vi "Main_Continuous.vi"() -> ()   [LabVIEW 2017]
doc: "This sample project is built upon the standard state machine template and shows how you could create an application that acquires, analyzes, and presents data. It includes functionality for presenting configuration dialogs, preserving settings between executions, loading and saving data, as well as exporting graph images and text files.\n\nIt is most appropriate for data that is acquired instantly as it does not allow for screen updates mid acquisition nor does it allow for continuous streaming to disk."
uses:
  controls/State.ctl
  controls/Data.ctl
  <vilib>/Utility/miscctls.llb/LVCursorListTypeDef.ctl
  <vilib>/Utility/miscctls.llb/LVAnnotationListTypeDef.ctl
  controls/UI References.ctl
  controls/HW Configuration.ctl
  controls/New Data Behavior.ctl
  controls/User Specified Data.ctl
  controls/Graph Data.ctl
  controls/Analysis Configuration.ctl
  subVIs/Settings Dialog.vi
  <extravilib>/ChannelInstances/Event Messenger-str.lvlib
  original/controls/Simulated Signal Type.ctl
  Program Files/National Instruments/LabVIEW 2017/examples/Data Communication/Protocols/TCP/TCP Multiple Connections/controls/TCP Multiple Connections State.ctl
  Program Files/National Instruments/LabVIEW 2017/examples/Data Communication/Protocols/TCP/TCP Multiple Connections/controls/TCP Multiple Connections Data.ctl
  <extravilib>/ChannelInstances/Event Messenger-c(a[.](str),t'Data.ctl').lvlib
  <extravilib>/ChannelInstances/Stream-t'Data.ctl'.lvlib
  controls/Signal Configuration.ctl
panel:
  out "# of Connections":i32
  in  "Settings":bool
  in  "Snapshot":bool
  in  "Analyze":bool
  in  "Clear":bool
  in  "Exit":bool
  in  "Acquire":bool
  in  "Export":bool
  in  "Save Data":bool
  in  "Load Data":bool
  out "Graph":waveform(dbl)[](graph)
  out "Status Bar":string
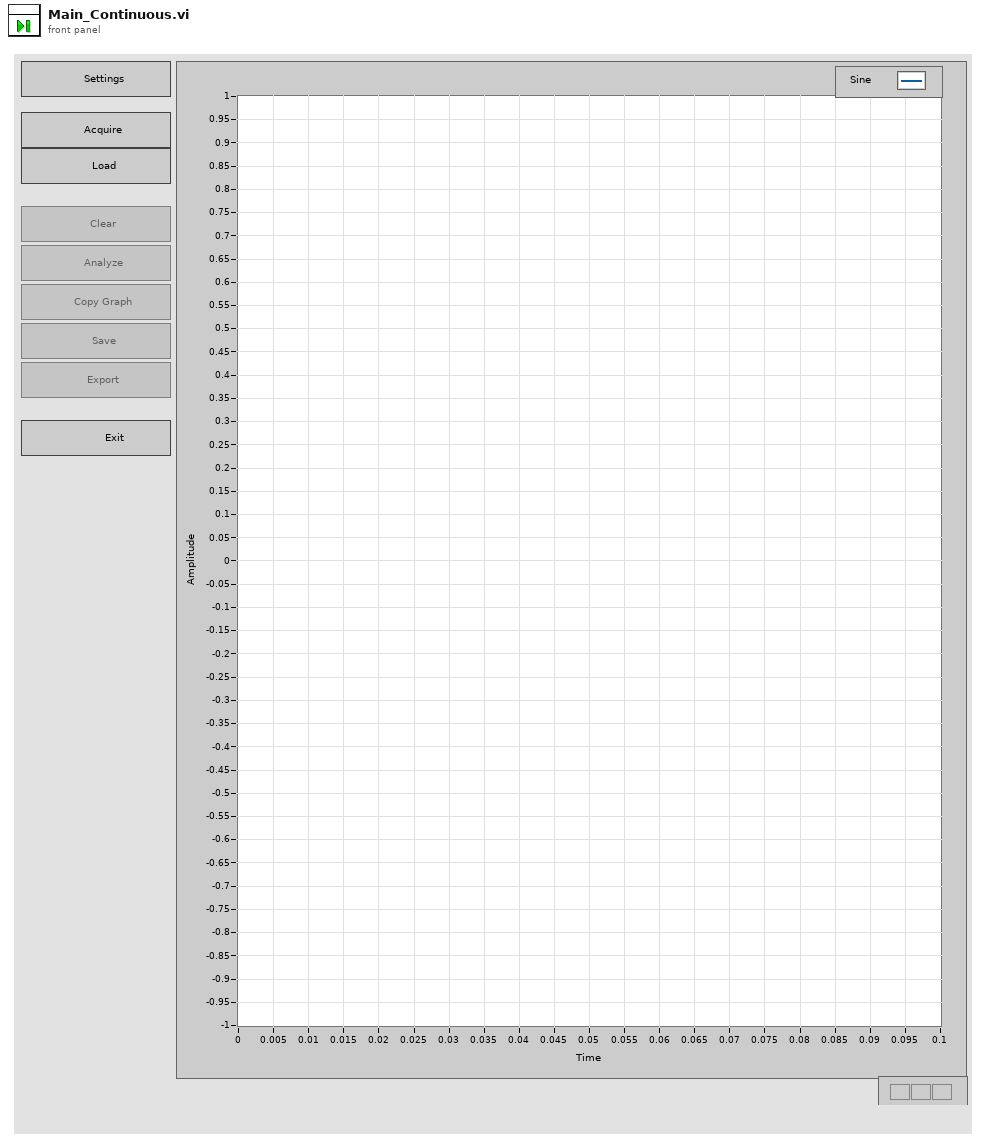
[diagram p1: front panel]
types:
  T1 = typedef "TCP Multiple Connections Data.ctl" = cluster{"Clients":refnum<k5>[], "Listener":refnum<k5>}
  T2 = typedef "TCP Multiple Connections State.ctl" = enum16{"Initialize", "Status Check", "Send Data", "Stop"}
  T3 = typedef "Data.ctl" = cluster{"UI References":T4, "Graph Data":T5, "User Specified":T8}
  T4 = typedef "UI References.ctl" = cluster{"Exit Ref":refnum<vi>, "Save Ref":refnum<vi>, "Open Ref":refnum<vi>, "Export Ref":refnum<vi>, "Acquire Ref":refnum<vi>, "Configure Ref":refnum<vi>, "Graph Ref":refnum<vi>, "Clear Ref":refnum<vi>, "Analyze Ref":refnum<vi>, "Status Ref":refnum<vi>, "Snapshot Ref":refnum<vi>}
  T5 = typedef "Graph Data.ctl" = cluster{"Data":waveform(dbl)[], "Annotation List":T6, "Cursor List":T7, "Analysis Data":waveform(dbl)[]}
  T6 = typedef "LVAnnotationListTypeDef.ctl" = cluster{"Name":string, "Color":u32, "Style":u8, "Point Style":u8, "Name Visible":bool, "Allow Drag":bool, "Annotation Mode":u32, "Plot":i32, "Index":i32, "Position":cluster{"X":dbl, "Y":dbl}, "X Scale":u32, "Y Scale":u32, "Show Arrow":bool, "Lock Name":bool, "Plot Area":i32, "Label Offset":cluster{"X":dbl, "Y":dbl}}[]
  T7 = typedef "LVCursorListTypeDef.ctl" = cluster{"Name":string, "Color":u32, "Style":u8, "Point Style":u8, "Name Visible":bool, "Allow Drag":bool, "Cursor Mode":u32, "Plot":i32, "Index":i32, "Position":cluster{"X":dbl, "Y":dbl}, "X Scale":u32, "Y Scale":u32, "Watch Plots":i32[], "Watch All Plots":bool, "Plot Area":i32, "Label Offset":cluster{"X":dbl, "Y":dbl}}[]
  T8 = typedef "User Specified Data.ctl" = cluster{"Hardware Configuration":T9, "Analysis Configuration":T11, "Signal Type":enum16{"Single Chirp", "From Excel"}, "New Data Behavior":T12, "Signal Configuration":T13}
  T9 = typedef "HW Configuration.ctl" = cluster{"Signal Channel":tag, "Response Channel":tag, "Trigger Channel":tag, "HW Refnum <Replace Me>":string, "Signal Type <Replace Me>":T10}
  T10 = typedef "Simulated Signal Type.ctl" = enum16{"Sine Wave", "Square Wave"}
  T11 = typedef "Analysis Configuration.ctl" = cluster{"Statistics":bool}
  T12 = typedef "New Data Behavior.ctl" = enum16{"Replace", "Overlay", "Append"}
  T13 = typedef "Signal Configuration.ctl" = cluster{"Chirp Amplitude":dbl, "I/O Limit":dbl, "Sample Rate":dbl, "Chirp Duration (s)":dbl, "Upper Frequency":dbl, "Lower Frequency":dbl, "Windowing":enum16{"None", "Exponential", "Flat top", "Hamming", "Hanning", "Kaiser-Bessel", "Rectangular"}}
  T14 = typedef "State.ctl" = enum16{"Initialize", "Wait for Event", "Update UI", "Configure", "Acquire", "Load Data", "Save Data", "Clear Data", "Export Data", "Analyze", "Copy Graph", "Exit"}
  T15 = enum16{"Standard", "Buffered", "CRLF", "Immediate"}
  T16 = typedef "Event Messenger-str.lvlib/))Channel.ctl" = refnum<queue>
  T17 = typedef "Event Messenger-c(a[.](str),t'Data.ctl').lvlib/))Channel.ctl" = refnum<queue>
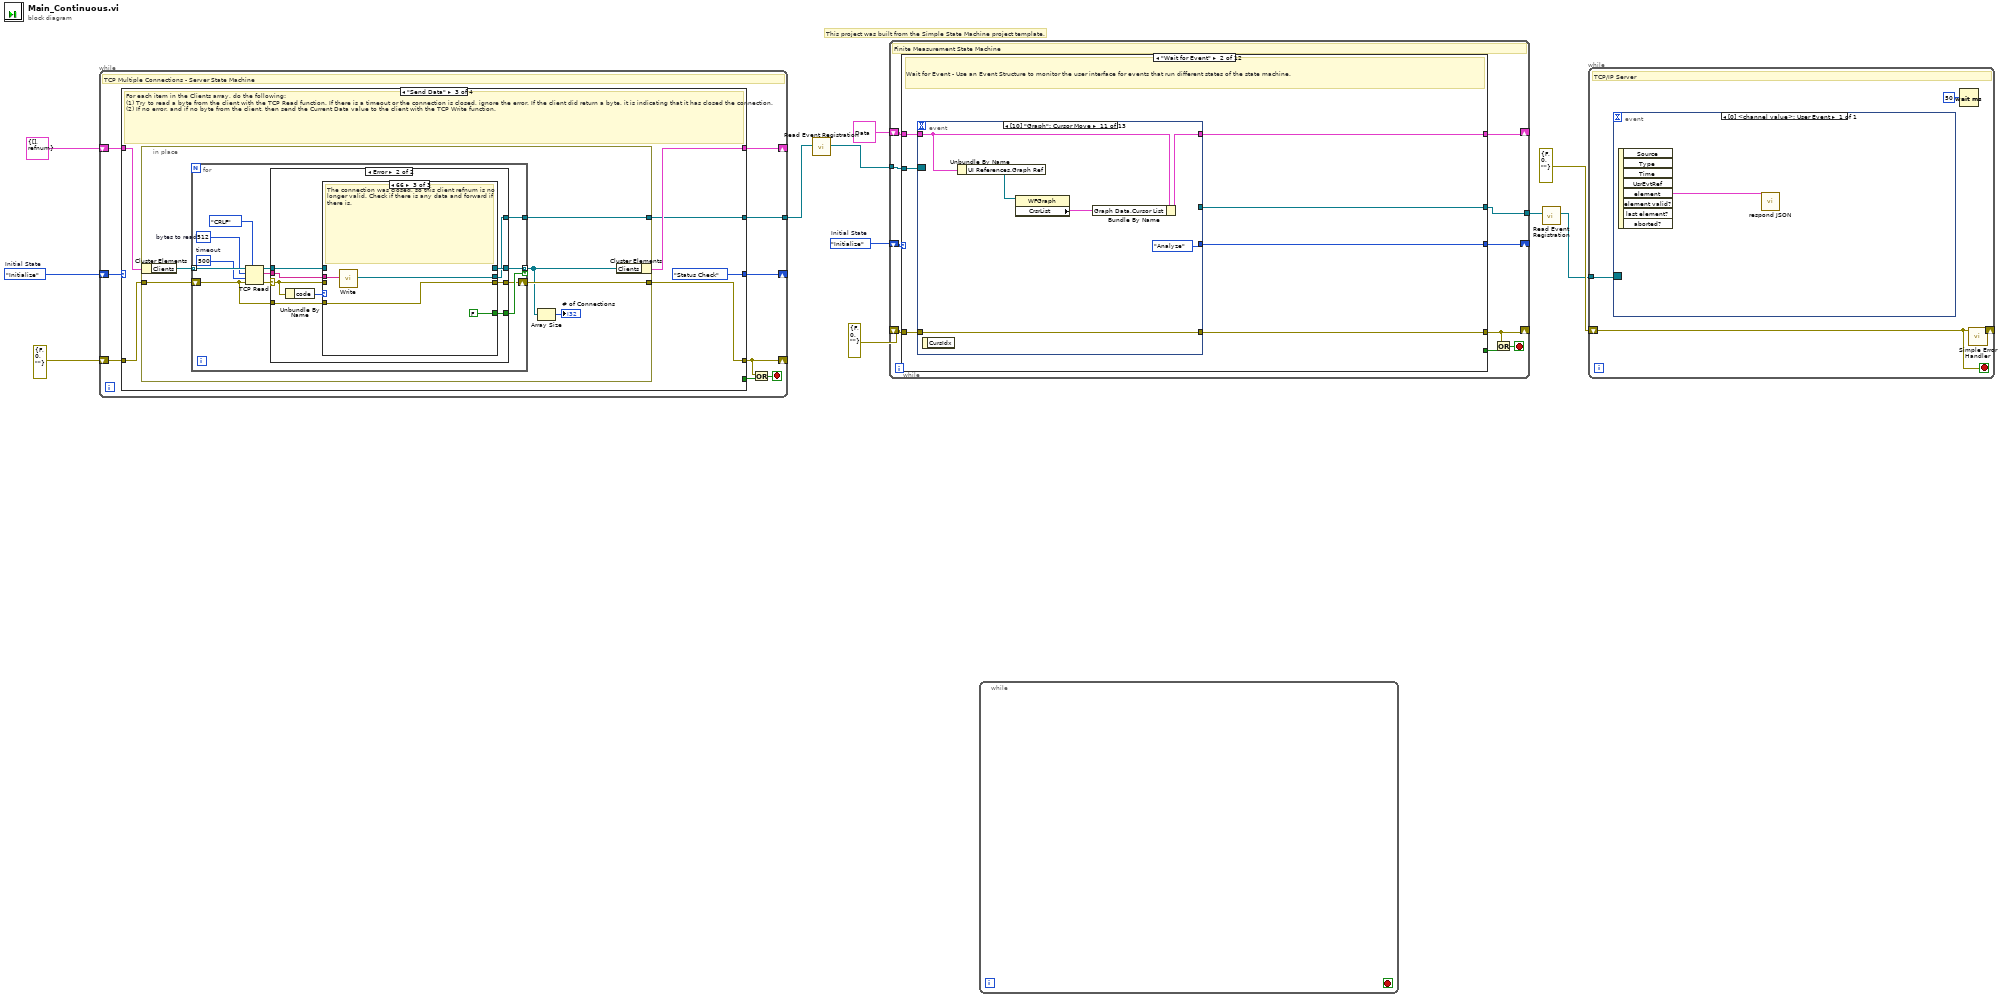
[diagram p0: block diagram]
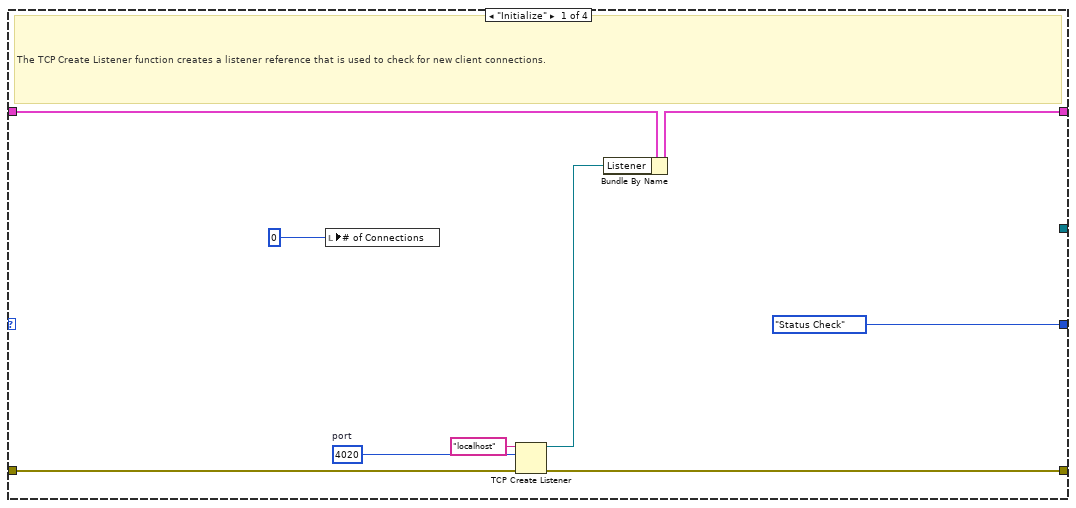
[diagram p2: hidden frame]
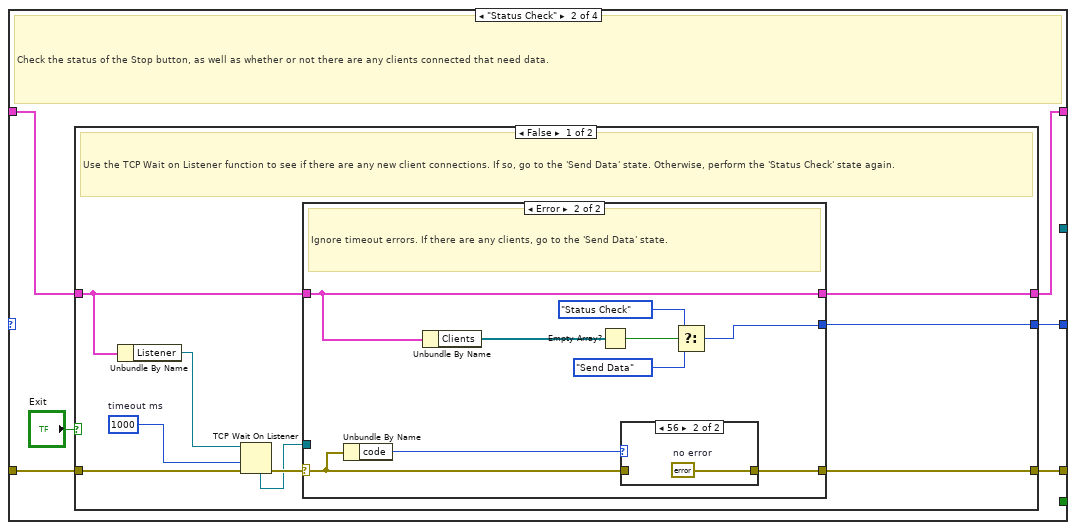
[diagram p3: hidden frame]
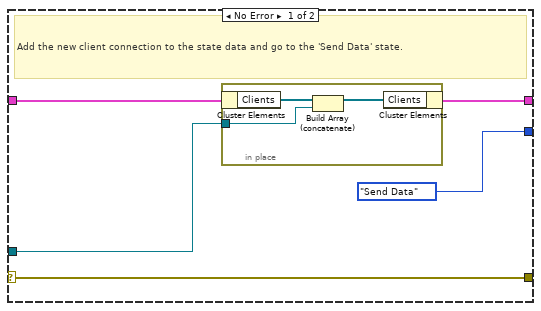
[diagram p4: hidden frame]
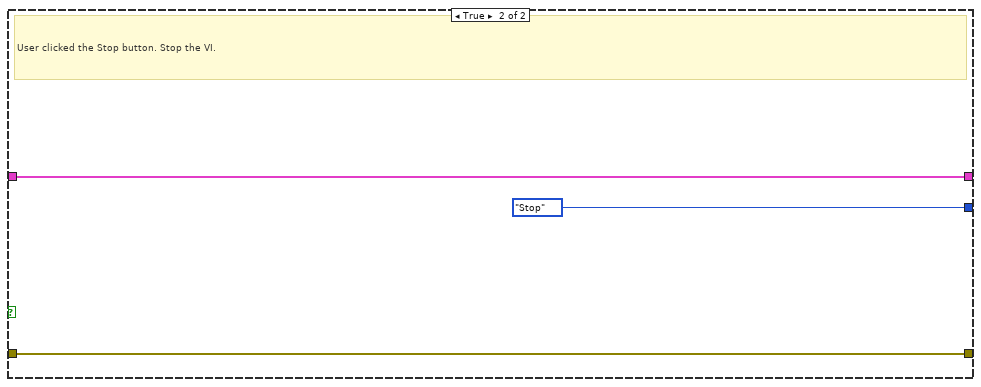
[diagram p6: hidden frame]
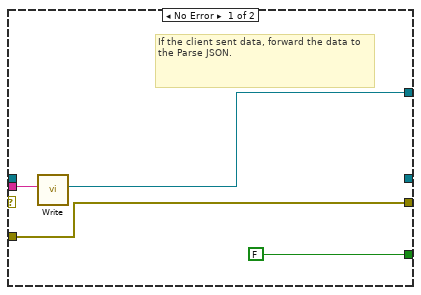
[diagram p7: hidden frame]
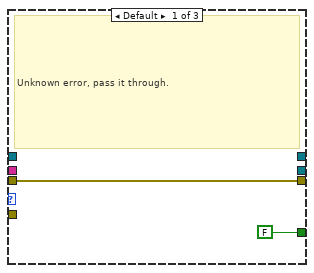
[diagram p8: hidden frame]
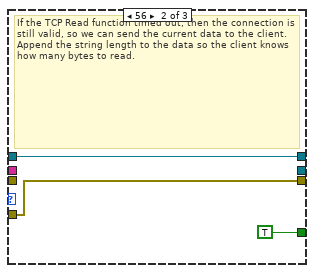
[diagram p9: hidden frame]
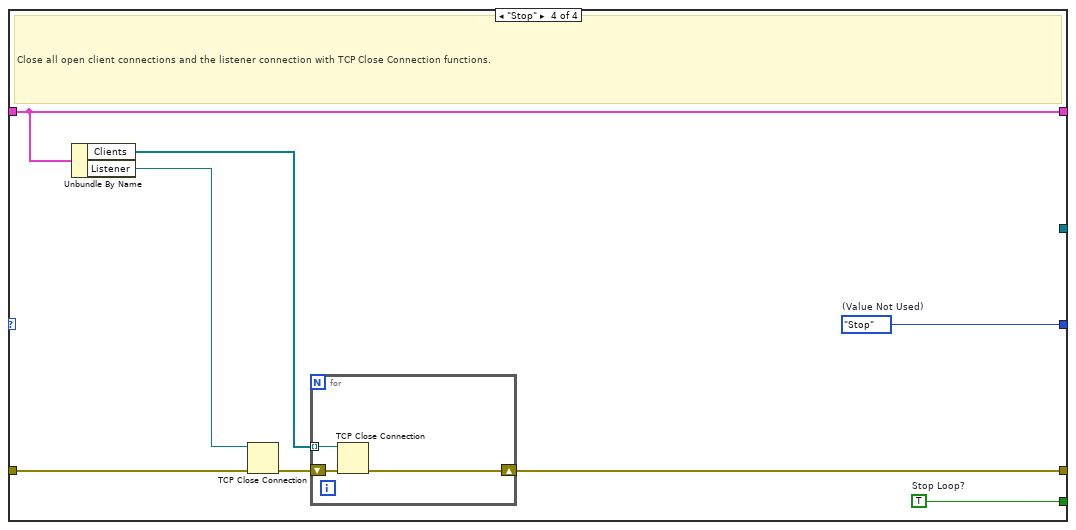
[diagram p10: hidden frame]
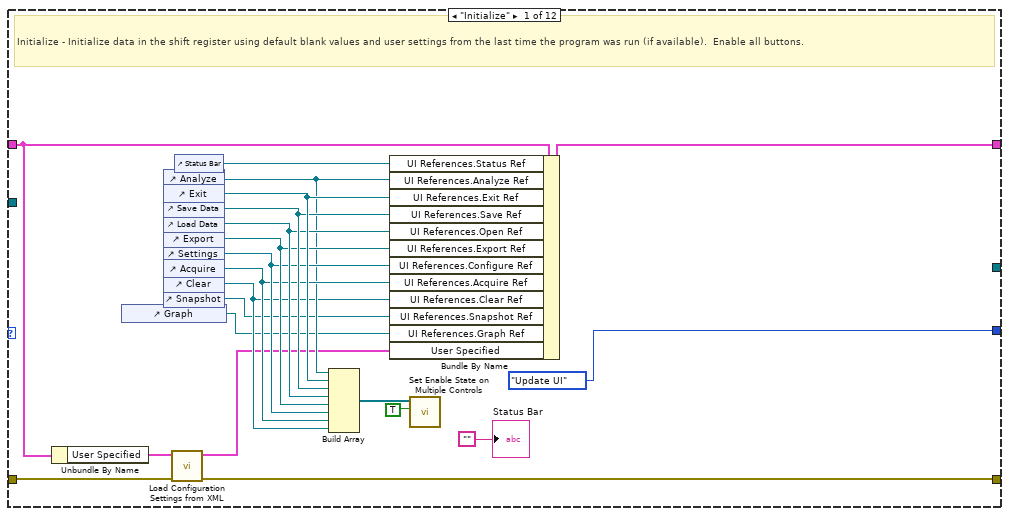
[diagram p11: hidden frame]
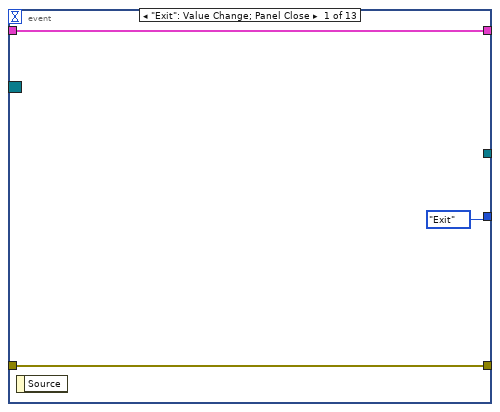
[diagram p12: hidden frame]
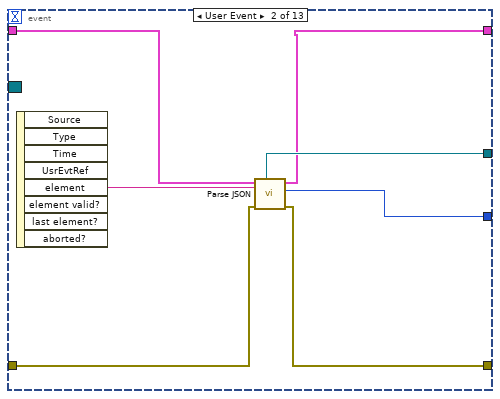
[diagram p13: hidden frame]
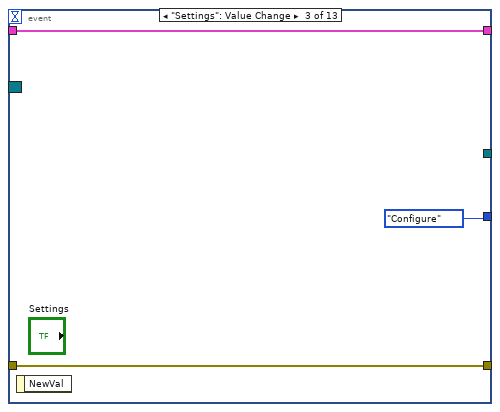
[diagram p14: hidden frame]
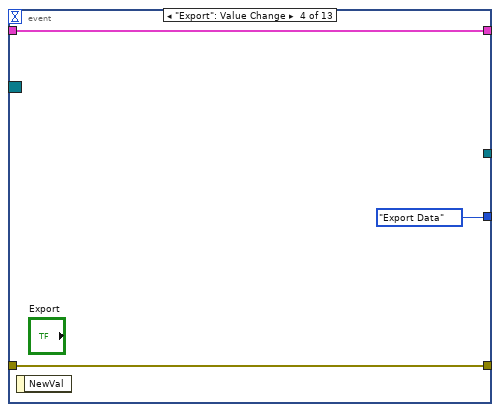
[diagram p15: hidden frame]
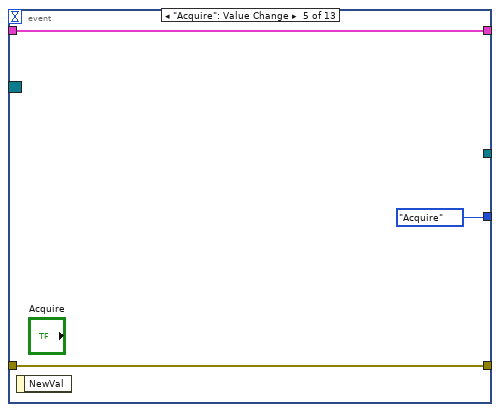
[diagram p16: hidden frame]
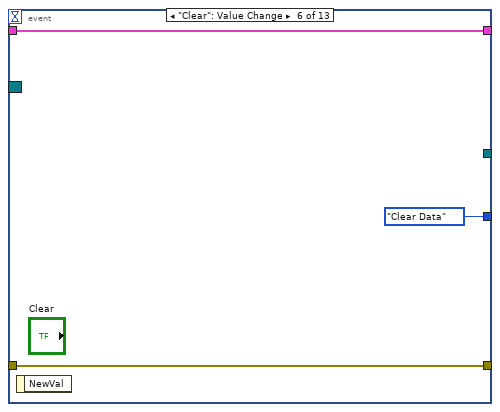
[diagram p17: hidden frame]
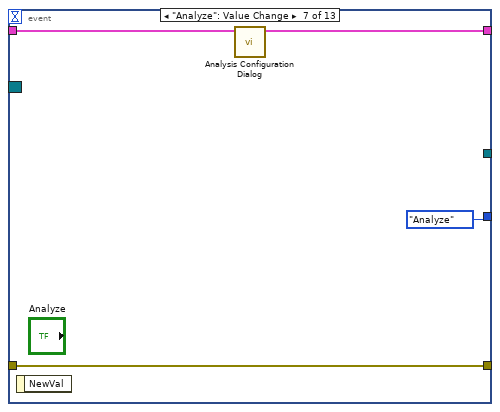
[diagram p18: hidden frame]
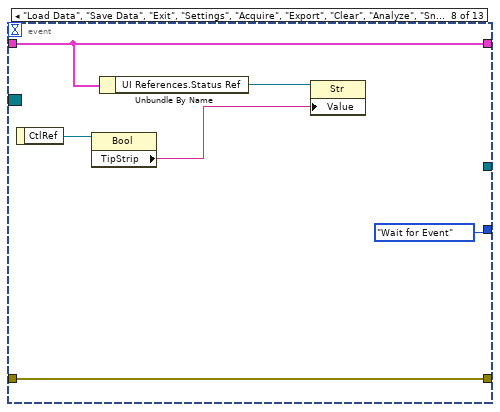
[diagram p19: hidden frame]
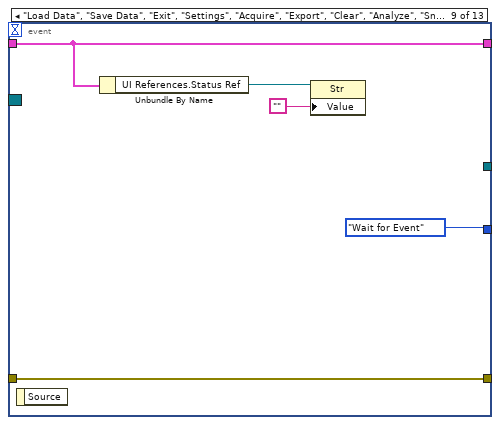
[diagram p20: hidden frame]
diagram:
  w4 = TCP_Multiple_Connections_State."Initialize"  # Initial State
  w11 = State."Initialize"  # Initial State
  # "This project was built from the Simple State Machine project template."
  n1 = while {
    shift-right: [w19] -> _
    shift-left: w4 -> [w20]
    shift-right: [w17] -> _
    shift-left: T1 {"Clients"=[], "Listener"=refnum} ("Data") -> [w18]
    shift-right: [w13] -> _
    shift-left: errorcluster {"status"=FALSE, "code"=0, "source"=""} ("error constant") -> [w16]
    tunnel: [w12] -> w1
    stop <- w14 stop-if-true
    # "TCP Multiple Connections - Server State Machine"
    n2 = case shown="\"Send Data\"" w20 {
      tunnel: [TCP_Multiple_Connections_State."Status Check" ("States") w35 TCP_Multiple_Connections_State."Status Check" ("States") w113] -> w19
      tunnel: [_ _ _ w120] -> w15
      tunnel: w18 -> [w27 w32 w70 w119]
      tunnel: [w26 w31 w69 w119] -> w17
      tunnel: w16 -> [w29 w34 w72 w118]
      tunnel: [w28 w33 w71 w116] -> w13
      tunnel: [_ _ w67 _] -> w12
      frame "Initialize" {
        w24 = u16 4020  # port
        # "The TCP Create Listener function creates a listener reference that is used to check for new client connections."
        n3 = local write "# of Connections"(0 ("Number of Client Connections")) -> ()
        n4 = TCP Create Listener(8:w29, 10:w24, 11:"localhost" ("service name")) -> (0:w28:errorcluster, 3:w25:refnum<k5>)  [unwired: 3 out]
        n5 = Bundle By Name(cluster=w27, "Listener"=w25) -> (w26:T1)
      }
      frame "Status Check" {
        # "Check the status of the Stop button, as well as whether or not there are any clients connected that need data."
        n6 = case shown="False" "Exit" {
          tunnel: [w44 TCP_Multiple_Connections_State."Stop" ("States")] -> w35
          tunnel: w34 -> [w43 w66]
          tunnel: [w36 w66] -> w33
          tunnel: w32 -> [w39 w65]
          tunnel: [w38 w65] -> w31
          frame False {
            w42 = 1000  # timeout ms
            # "Use the TCP Wait on Listener function to see if there are any new client connections. If so, go to the 'Send Data' state. Otherwise, perform the 'Status Check' state again."
            n7 = Unbundle By Name(w39) -> ("Listener"=w37:refnum<k5>)
            n8 = TCP Wait On Listener(8:w43, 9:w42, 11:w37) -> (0:w41:errorcluster, 4:w40:refnum<k5>)  [unwired: 4 out]
            n9 = case shown="Error" w41 {
              selector: w41 -> [w47 w61]
              tunnel: [TCP_Multiple_Connections_State."Send Data" ("States") w55] -> w44
              tunnel: w40 -> [w48 _]
              tunnel: w39 -> [w49 w58]
              tunnel: [w46 w58] -> w38
              tunnel: [w47 w59] -> w36
              frame No Error {
                # "Add the new client connection to the state data and go to the 'Send Data' state."
                n10 = in-place {
                  in-place-border: w48 -> [w50]
                  n11 = in-place-cluster #1(w49) -> ("Clients"=w52:refnum<k5>[])
                  n12 = Build Array (concatenate)(w52, w50) -> (w51:refnum<k5>[])
                  n13 = in-place-cluster #1("Clients"=w51) -> (w46:T1)
                }
              }
              frame Error {
                # "Ignore timeout errors. If there are any clients, go to the 'Send Data' state."
                n14 = Unbundle By Name(w61) -> ("code"=w60:i32)
                n15 = Unbundle By Name(w58) -> ("Clients"=w57:refnum<k5>[])
                n16 = Empty Array?(array=w57) -> (empty?=w56:bool)
                n17 = case shown="56" w60 {
                  tunnel: w61 -> [w62 _]
                  tunnel: [w62 w63] -> w59
                  frame Default {
                  }
                  frame 56 {
                    w63 = errorcluster {"status"=FALSE, "code"=0, "source"=""}  # no error
                  }
                }
                n18 = Select(t=TCP_Multiple_Connections_State."Status Check" ("States"), s=w56, f=TCP_Multiple_Connections_State."Send Data" ("States")) -> (s? t:f=w55:T2)
              }
            }
          }
          frame True {
            # "User clicked the Stop button. Stop the VI."
          }
        }
      }
      frame "Send Data" {
        # "For each item in the Clients array, do the following:\n(1) Try to read a byte from the client with the TCP Read function. If there is a timeout or the connection is closed, ignore the error. If the client did return a byte, it is indicating that it has closed the connection.\n(2) If no error, and if no byte from the client, then send the Current Data value to the client with the TCP Write function."
        n19 = in-place {
          in-place-border: w72 -> [w78]
          in-place-border: [w77] -> w71
          in-place-border: [w73] -> w67
          n20 = in-place-cluster #2(w70) -> ("Clients"=w75:refnum<k5>[])
          n21 = for {
            tunnel: w75 -> [w90] mode=indexing
            shift-right: [w82] -> w77
            shift-left: w78 -> [w81]
            tunnel: [w84] -> w74 mode=indexing if=w83
            tunnel: [w79] -> w73
            w87 = 500  # timeout
            w88 = 512  # bytes to read
            n22 = TCP Read(connection ID=w90, bytes to read=w88, error in (no error)=w81, 7:T15."CRLF" ("mode (standard)"), 9:w87) -> (connection ID out=w89:refnum<k5>, data out=w85:string, error out=w86:errorcluster)
            n23 = case shown="Error" w86 {
              selector: w86 -> [_ w102]
              tunnel: w89 -> [_ w99]
              tunnel: w85 -> [w93 w96]
              tunnel: [_ w97] -> w84
              tunnel: [FALSE w98] -> w83
              tunnel: [w91 w101] -> w82
              tunnel: w81 -> [w91 w100]
              tunnel: [w92 w95] -> w79
              frame No Error {
                # "If the client sent data, forward the data to the Parse JSON."
                # "If the client sent data, it is saying that the connection should be closed."
                n24 = call <extravilib>:"Write.vi"("element"=w93) -> ("channel"=w92:T16)  [unwired: 9 in, 1 out]
              }
              frame Error {
                # "Ignore connection closed and timeout errors"
                n25 = Unbundle By Name(w102) -> ("code"=w103:i32)
                n26 = case shown="66" w103 {
                  tunnel: w102 -> [w105 _ _]
                  tunnel: [w105 w106 w112] -> w101
                  tunnel: w100 -> [_ w106 w112]
                  tunnel: w99 -> [_ w108 _]
                  tunnel: [FALSE TRUE FALSE] -> w98
                  tunnel: [_ w108 _] -> w97
                  tunnel: w96 -> [_ _ w110]
                  tunnel: [_ _ w109] -> w95
                  frame Default {
                    # "Unknown error, pass it through."
                  }
                  frame 56 {
                    # "If the TCP Read function timed out, then the connection is still valid, so we can send the current data to the client. Append the string length to the data so the client knows how many bytes to read."
                  }
                  frame 66 {
                    # "The connection was closed, so this client refnum is no longer valid. Check if there is any data and forward if there is."
                    n27 = call <extravilib>:"Write.vi"("element"=w110) -> ("channel"=w109:T16)  [unwired: 9 in, 1 out]
                  }
                }
              }
            }
          }
          n28 = Array Size(array=w74) -> (size(s)=→"# of Connections":i32)
          n29 = in-place-cluster #2("Clients"=w74) -> (w69:T1)
        }
      }
      frame "Stop" {
        w113 = TCP_Multiple_Connections_State."Stop"  # (Value Not Used)
        w120 = TRUE  # Stop Loop?
        # "Close all open client connections and the listener connection with TCP Close Connection functions."
        n30 = Unbundle By Name(w119) -> ("Clients"=w117:refnum<k5>[], "Listener"=w114:refnum<k5>)
        n31 = TCP Close Connection(connection ID=w114, error in (no error)=w118) -> (error out=w115:errorcluster)  [unwired: 1 in, 1 out]
        n32 = for {
          shift-right: [w122] -> w116
          shift-left: w115 -> [w123]
          tunnel: w117 -> [w121] mode=indexing
          n33 = TCP Close Connection(connection ID=w121, error in (no error)=w123) -> (error out=w122:errorcluster)  [unwired: 1 in, 1 out]
        }
      }
    }
    n34 = Or(x=w13, y=w15) -> (x .or. y?=w14:bool)
  }
  n35 = call <extravilib>:"Read Event Registration.vi"("channel"=w1) -> ("event registration refnum"=w9:refnum<event-registration>)  [unwired: 10 in]
  n36 = while {
    shift-right: [w125] -> _
    shift-left: w11 -> [w133]
    shift-right: [w131] -> _
    shift-left: T3 {"UI References"={"Exit Ref"=refnum, "Save Ref"=refnum, "Open Ref"=refnum, "Export Ref"=refnum, "Acquire Ref"=refnum, "Configure Ref"=refnum, "Graph Ref"=refnum, "Clear Ref"=refnum, "Analyze Ref"=refnum, "Status Ref"=refnum, "Snapshot Ref"=refnum}, "Graph Data"={"Data"=[], "Annotation List"=[], "Cursor List"=[], "Analysis Data"=[]}, "User Specified"={"Hardware Configuration"={"Signal Channel"="", "Response Channel"="", "Trigger Channel"="", "HW Refnum <Replace Me>"="", "Signal Type <Replace Me>"=enum."Sine Wave"}, "Analysis Configuration"={"Statistics"=TRUE}, "Signal Type"=enum."Single Chirp", "New Data Behavior"=enum."Replace", "Signal Configuration"={"Chirp Amplitude"=0.1, "I/O Limit"=10.0, "Sample Rate"=1000000.0, "Chirp Duration (s)"=0.01, "Upper Frequency"=0.0, "Lower Frequency"=0.0, "Windowing"=enum."None"}}} ("Data") -> [w132]
    shift-right: [w128] -> _
    shift-left: errorcluster {"status"=FALSE, "code"=0, "source"=""} ("error constant") -> [w130]
    tunnel: w9 -> [w127]
    tunnel: [w126] -> w6
    stop <- w124 stop-if-true
    # "Finite Measurement State Machine"
    n37 = case shown="\"Wait for Event\"" w133 {
      tunnel: [_ w161 _ _ _ _ _ _ _ _ _ _] -> w126
      tunnel: [_ _ _ _ _ _ _ _ _ _ _ w321] -> w129
      tunnel: w132 -> [w146 w160 w229 w241 w242 w267 w281 w293 w304 w307 w313 w319]
      tunnel: [w154 w159 w229 w240 w249 w262 w281 w293 w303 w307 w313 w319] -> w131
      tunnel: w130 -> [w144 w158 w231 w239 w250 w266 w283 w296 w305 w308 w312 w316]
      tunnel: [w143 w157 w231 w238 w250 w265 w279 w290 w305 w308 w311 w315] -> w128
      tunnel: w127 -> [_ w156 _ _ _ _ _ _ _ _ _ _]
      tunnel: [State."Update UI" ("Next State") w155 State."Wait for Event" ("(Value Not Used)") w232 State."Update UI" ("Next State") State."Update UI" ("(Value Not Used)") State."Wait for Event" ("(Value Not Used)") State."Wait for Event" ("(Value Not Used)") State."Update UI" ("(Value Not Used)") State."Update UI" ("(Value Not Used)") State."Wait for Event" ("(Value Not Used)") w314] -> w125
      frame "Initialize" {
        # "Initialize - Initialize data in the shift register using default blank values and user settings from the last time the program was run (if available).  Enable all buttons."
        n38 = Unbundle By Name(w146) -> ("User Specified"=w145:T8)
        n39 = control-ref of="Graph"() -> (w135:refnum<vi>)
        n40 = control-ref of="Analyze"() -> (w142:refnum<vi>)
        n41 = control-ref of="Exit"() -> (w153:refnum<vi>)
        n42 = control-ref of="Save Data"() -> (w152:refnum<vi>)
        n43 = control-ref of="Load Data"() -> (w151:refnum<vi>)
        n44 = control-ref of="Export"() -> (w150:refnum<vi>)
        n45 = control-ref of="Settings"() -> (w149:refnum<vi>)
        n46 = control-ref of="Acquire"() -> (w148:refnum<vi>)
        n47 = control-ref of="Clear"() -> (w140:refnum<vi>)
        n48 = control-ref of="Snapshot"() -> (w136:refnum<vi>)
        n49 = call "Load Configuration Settings from XML.vi"("error in (no error)"=w144, "User Configuration in"=w145) -> ("error out"=w143:errorcluster, "User Configuration out"=w138:T8)  [unwired: 8 in]
        n50 = control-ref of="Status Bar"() -> (w141:refnum<vi>)
        n51 = Build Array(w142, w153, w152, w151, w150, w149, w148, w140) -> (w147:refnum<vi>[])
        n52 = Bundle By Name(cluster=w146, "UI References.Status Ref"=w141, "UI References.Analyze Ref"=w142, "UI References.Exit Ref"=w153, "UI References.Save Ref"=w152, "UI References.Open Ref"=w151, "UI References.Export Ref"=w150, "UI References.Configure Ref"=w149, "UI References.Acquire Ref"=w148, "UI References.Clear Ref"=w140, "UI References.Snapshot Ref"=w136, "UI References.Graph Ref"=w135, "User Specified"=w138) -> (w154:T3)
        n53 = call "Set Enable State on Multiple Controls.vi"("Enable?"=TRUE, "Controls"=w147) -> ()  [unwired: 10 in]
        "Status Bar" <- "" ("Status Bar")
      }
      frame "Wait for Event" {
        # "Wait for Event - Use an Event Structure to monitor the user interface for events that run different states of the state machine."
        n54 = event shown="[10] \"Graph\": Cursor Move" {
          selector: w156 -> [_ _ _ _ _ _ _ _ _ _ _ _ _]
          dyn-events: _ -> [_ _ _ _ _ _ _ _ _ _ _ _ _]
          timeout: _ -> [_ _ _ _ _ _ _ _ _ _ _ _ _]
          tunnel: [_ w167 _ _ _ _ _ _ _ _ _ _ _] -> w161
          tunnel: w160 -> [w164 w170 w174 w177 w180 w183 w186 w191 w197 w201 w203 w210 w213]
          tunnel: [w164 w165 w174 w177 w180 w183 w185 w191 w197 w201 w206 w210 w213] -> w159
          tunnel: w158 -> [w163 w169 w173 w176 w179 w182 w187 w193 w198 w200 w207 w209 w212]
          tunnel: [w163 w168 w173 w176 w179 w182 w187 w193 w198 w200 w207 w209 w212] -> w157
          tunnel: [State."Exit" ("Next State") w166 State."Configure" ("Next State") State."Export Data" ("Next State") State."Acquire" ("Next State") State."Clear Data" ("Next State") State."Analyze" ("Next State") State."Wait for Event" ("Next State") State."Wait for Event" ("Next State") State."Copy Graph" ("Next State") State."Analyze" ("Next State") State."Load Data" ("Next State") State."Save Data" ("Next State")] -> w155
          event "Exit": Value Change; Panel Close {
            n55 = event-data() -> ()  [unwired: 1 in, 1 out]
          }
          event User Event {
            n56 = event-data() -> ("element"=w171:string)  [unwired: 1 in, 7 out]
            n57 = call "Parse JSON.vi"("error in (no error)"=w169, "element"=w171, "Data In"=w170) -> ("error out"=w168:errorcluster, "States"=w166:T14, "Data Out"=w165:T3, "channel"=w167:T17)  [unwired: 3 in]
          }
          event "Settings": Value Change {
            n58 = event-data() -> ()  [unwired: 1 in, 1 out]
          }
          event "Export": Value Change {
            n59 = event-data() -> ()  [unwired: 1 in, 1 out]
          }
          event "Acquire": Value Change {
            n60 = event-data() -> ()  [unwired: 1 in, 1 out]
          }
          event "Clear": Value Change {
            n61 = event-data() -> ()  [unwired: 1 in, 1 out]
          }
          event "Analyze": Value Change {
            n62 = event-data() -> ()  [unwired: 1 in, 1 out]
            n63 = call "Analysis Configuration Dialog.vi"("Data in"=w186) -> ("Data out"=w185:T3)  [unwired: 10 in]
          }
          event "Load Data", "Save Data", "Exit", "Settings", "Acquire", "Export", "Clear", "Analyze", "Snapshot": Mouse Enter {
            n64 = event-data() -> ("CtlRef"=w192:refnum<vi>)  [unwired: 1 in]
            n65 = property class="Bool"(reference=w192) -> ("TipStrip"=w189:string)  [unwired: 1 in, 2 out]
            n66 = Unbundle By Name(w191) -> ("UI References.Status Ref"=w190:refnum<vi>)
            n67 = property class="Str"(reference=w190, "Value"=w189) -> ()  [unwired: 1 in, 2 out]
          }
          event "Load Data", "Save Data", "Exit", "Settings", "Acquire", "Export", "Clear", "Analyze", "Snapshot": Mouse Leave {
            n68 = event-data() -> ()  [unwired: 1 in, 1 out]
            n69 = Unbundle By Name(w197) -> ("UI References.Status Ref"=w196:refnum<vi>)
            n70 = property class="Str"(reference=w196, "Value"="") -> ()  [unwired: 1 in, 2 out]
          }
          event "Snapshot": Value Change {
            n71 = event-data() -> ()  [unwired: 1 in, 1 out]
          }
          event "Graph": Cursor Move {
            n72 = event-data() -> ()  [unwired: 1 in, 1 out]
            n73 = Unbundle By Name(w203) -> ("UI References.Graph Ref"=w205:refnum<vi>)
            n74 = property class="WFGraph"(reference=w205) -> ("CrsrList"=w204:T7)  [unwired: 1 in, 2 out]
            n75 = Bundle By Name(cluster=w203, "Graph Data.Cursor List"=w204) -> (w206:T3)
          }
          event "Load Data": Value Change {
            n76 = event-data() -> ()  [unwired: 1 in, 1 out]
          }
          event "Save Data": Value Change {
            n77 = event-data() -> ()  [unwired: 1 in, 1 out]
          }
        }
      }
      frame "Update UI" {
        # "These buttons should be disabled when there is no data visible."
        # "Update UI - Update the graph using the waveform data stored in the shift register.  If there is no data to display disable buttons that act on the current data."
        n78 = Unbundle By Name(w229) -> ("Graph Data.Data"=w225:waveform(dbl)[], "Graph Data.Analysis Data"=w215:waveform(dbl)[], "Graph Data.Annotation List"=w230:T6, "Graph Data.Cursor List"=w226:T7)
        n79 = Unbundle By Name(w229) -> ("UI References.Clear Ref"=w221:refnum<vi>, "UI References.Analyze Ref"=w220:refnum<vi>, "UI References.Save Ref"=w228:refnum<vi>, "UI References.Export Ref"=w218:refnum<vi>, "UI References.Snapshot Ref"=w219:refnum<vi>)
        n80 = Build Array (concatenate)(w225, w215) -> (w223:waveform(dbl)[])
        "Graph" <- w223
        n81 = Array Size(array=w223) -> (size(s)=w224:i32)
        n82 = Not Equal To 0?(x=w224) -> (x != 0?=w222:bool)
        n83 = call "Get Scale Labels.vi"("Array of Waveforms"=w223) -> ("Y Scale Label Text"=w216:string, "X Scale Label Text"=w217:string)  [unwired: 9 in]
        n84 = Build Array(w221, w220, w228, w218, w219) -> (w227:refnum<vi>[])
        n85 = property on="Graph" class="WFGraph (strict)"("AnntList"=w230, "CrsrList"=w226, "LegNumRows"=w224, "XScale.NameLbl.Text"=w217, "YScale.NameLbl.Text"=w216) -> ()  [unwired: 2 in, 2 out]
        n86 = call "Set Enable State on Multiple Controls.vi"("Enable?"=w222, "Controls"=w227) -> ()  [unwired: 10 in]
      }
      frame "Configure" {
        # "Configure - Spawns a dialog that allows the user to set any user configurable settings."
        n87 = Unbundle By Name(w241) -> ("User Specified"=w234:T8)
        n88 = call-by-ref "?"("error in (no error)"=w239, "Configuration in"=w234) -> ("error out"=w238:errorcluster, "UI Refresh Needed?"=w237:bool, "Configuration out"=w233:T8)  [unwired: 9 in, 2 out]
        n89 = Bundle By Name(cluster=w241, "User Specified"=w233) -> (w240:T3)
        n90 = Select(t=State."Update UI" ("Next State if true"), s=w237, f=State."Wait for Event" ("Next State if false")) -> (s? t:f=w232:T14)
      }
      frame "Acquire" {
        # "Acquire - Uses the current hardware configuration to acquire a new data set and stores it in the state data."
        n91 = Unbundle By Name(w242) -> ("UI References.Status Ref"=w244:refnum<vi>, "User Specified.Hardware Configuration"=w248:T9)
        n92 = call "Acquire Data from Hardware.vi"("Hardware Configuration"=w248) -> ("error out"=w245:errorcluster, "Graph Data"=w246:waveform(dbl)[])  [unwired: 9 in]
        n93 = case shown="Error" w245 {
          selector: w245 -> [w253 w258]
          tunnel: [w256 _] -> w243
          tunnel: [w255 _] -> _
          tunnel: w246 -> [w254 _]
          tunnel: ["Data acquired." ("Data acquired") "Data not acquired." ("Data not acquired")] -> w247
          frame No Error {
            n94 = call "Incorporate New Data.vi"("error in (no error)"=w253, "New Graph Data"=w254) -> ("error out"=w255:errorcluster, "Data out"=w256:T3)  [unwired: 8 in]
          }
          frame Error {
            n95 = call <vilib>:"Simple Error Handler.vi"("error in (no error)"=w258) -> ()  [unwired: 4 in, 5 out]
          }
        }
        n96 = property class="Str"(reference=w244, "Value"=w247) -> ()  [unwired: 1 in, 2 out]
        n97 = call <extravilib>:"Write.vi"("element"=w243) -> ()  [unwired: 8 in, 3 out]
        n98 = call <extravilib>:"Read.vi"() -> ("element"=w249:T3)  [unwired: 7 in, 4 out]
      }
      frame "Load Data" {
        # "Load Data - Loads data from a TDMS file and incorporates it with the existing data according to the user's preference."
        n99 = call "Load Data.vi"("error in (no error)"=w266) -> ("error out"=w264:errorcluster, "New Graph Data"=w261:waveform(dbl)[])  [unwired: 9 in]
        n100 = case shown="No Error" w264 {
          selector: w264 -> [w270 w275]
          tunnel: w267 -> [w269 w276]
          tunnel: [w273 w276] -> w262
          tunnel: [w272 _] -> w265
          tunnel: w261 -> [w271 _]
          tunnel: ["Data loaded." ("Data loaded") "Data not loaded." ("Data not loaded")] -> w263
          frame No Error {
            n101 = call "Incorporate New Data.vi"("error in (no error)"=w270, "New Graph Data"=w271, "Data in"=w269) -> ("error out"=w272:errorcluster, "Data out"=w273:T3)  [unwired: 7 in]
          }
          frame Error {
            n102 = call <vilib>:"Simple Error Handler.vi"("error in (no error)"=w275) -> ()  [unwired: 4 in, 5 out]
          }
        }
        n103 = Unbundle By Name(w262) -> ("UI References.Status Ref"=w260:refnum<vi>)
        n104 = property class="Str"(reference=w260, "Value"=w263) -> ()  [unwired: 1 in, 2 out]
      }
      frame "Save Data" {
        # "Save Data - Saves the existing measurement data to a TDMS file."
        n105 = Unbundle By Name(w281) -> ("UI References.Status Ref"=w280:refnum<vi>, "Graph Data.Data"=w284:waveform(dbl)[])
        n106 = call "Save Data.vi"("error in (no error)"=w283, "Data"=w284) -> ("error out"=w282:errorcluster)  [unwired: 9 in]
        n107 = case shown="No Error" w282 {
          selector: w282 -> [w285 w288]
          tunnel: ["Data saved." ("Data saved") "Data not saved." ("Data not saved")] -> w278
          tunnel: [w285 _] -> w279
          frame No Error {
          }
          frame Error {
            n108 = call <vilib>:"Simple Error Handler.vi"("error in (no error)"=w288) -> ()  [unwired: 4 in, 5 out]
          }
        }
        n109 = property class="Str"(reference=w280, "Value"=w278) -> ()  [unwired: 1 in, 2 out]
      }
      frame "Export Data" {
        # "Export Data - Exports the currently loaded measurement and analysis data to a text file that can be imported into a spreadsheet or other application."
        n110 = Unbundle By Name(w293) -> ("UI References.Status Ref"=w291:refnum<vi>, "Graph Data"=w292:T5)
        n111 = call "Export Data.vi"("error in (no error)"=w296, "Graph Data"=w292) -> ("error out"=w294:errorcluster)  [unwired: 9 in]
        n112 = case shown="No Error" w294 {
          selector: w294 -> [w297 w300]
          tunnel: ["Data exported." ("Data exported") "Data not exported." ("Data not exported")] -> w295
          tunnel: [w297 _] -> w290
          frame No Error {
          }
          frame Error {
            n113 = call <vilib>:"Simple Error Handler.vi"("error in (no error)"=w300) -> ()  [unwired: 4 in, 5 out]
          }
        }
        n114 = property class="Str"(reference=w291, "Value"=w295) -> ()  [unwired: 1 in, 2 out]
      }
      frame "Clear Data" {
        # "Clear Data - Clears the data currently in the graph."
        n115 = Bundle By Name(cluster=w304, "Graph Data"=T5 {"Data"=[], "Annotation List"=[], "Cursor List"=[], "Analysis Data"=[]} ("Graph")) -> (w303:T3)
      }
      frame "Analyze" {
        # "#CodeRecommended - Add your own signal analysis here."
        # "Analyze - Analyzes the measurement data."
        n116 = Unbundle By Name(w307) -> ("Graph Data"=w309:T5)
        n117 = call "Statistical Analysis.vi"("Graph Data In"=w309) -> ()  [unwired: 9 in, 2 out]
      }
      frame "Copy Graph" {
        # "Copy Graph - Places an image of the graph on the clipboard for pasting into reports or emails."
        n118 = call "Copy Graph to Clipboard.vi"("error in (no error)"=w312, "Graph Data"=w313) -> ("error out"=w311:errorcluster)  [unwired: 9 in]
      }
      frame "Exit" {
        w321 = TRUE  # Stop Loop?
        w314 = State."Exit"  # (Value Not Used)
        # "Exit - Saves the user's settings to an XML file and stops execution."
        n119 = Unbundle By Name(w319) -> ("UI References.Status Ref"=w317:refnum<vi>, "User Specified"=w320:T8)
        n120 = call "Save Configuration Settings to XML.vi"("error in (no error)"=w316, "User Configuration"=w320) -> ("error out"=w315:errorcluster)  [unwired: 9 in]
        n121 = property class="Str"(reference=w317, "Value"="Application exit." ("Stopped")) -> ()  [unwired: 1 in, 2 out]
      }
    }
    n122 = Or(x=w128, y=w129) -> (x .or. y?=w124:bool)
  }
  n123 = while {
    stop <- _ stop-if-true
  }
  n124 = call <extravilib>:"Read Event Registration.vi"("channel"=w6) -> ("event registration refnum"=w5:refnum<event-registration>)  [unwired: 10 in]
  n125 = while {
    shift-right: [w322] -> _
    shift-left: errorcluster {"status"=FALSE, "code"=0, "source"=""} ("error constant") -> [w322]
    tunnel: w5 -> [w324]
    stop <- w322 stop-if-true
    # "TCP/IP Server"
    n126 = event shown="[0] <channel value>: User Event" {
      selector: w324 -> [_]
      dyn-events: _ -> [_]
      timeout: _ -> [_]
      event User Event {
        n127 = event-data() -> ("element"=w325:cluster{string[], "Data In 2":T3})  [unwired: 1 in, 7 out]
        n128 = call "respond JSON.vi"("Message In"=w325) -> ()  [unwired: 11 in]
      }
    }
    n129 = Wait (ms)(milliseconds to wait=u32 50) -> ()  [unwired: 1 out]
  }
  n130 = call <vilib>:"Simple Error Handler.vi"() -> ()  [unwired: 5 in, 5 out]
